vi "循环的使用.vi"() -> ()   [LabVIEW 2018]
panel:
  out "布尔":bool
  out "平均值":dbl
  # "创建一个VI，产生50个随机数，并采用循环结构求得这50个随机数的平均值，\n将平均值显示出来，再对平均值的范围进行判断，如果在0.6-0.9范围内，则\n点亮指示灯，否则知识点熄灭，并计算程序运行所消耗的时间。"
  # "20174080221\n王靖\n电子二班"
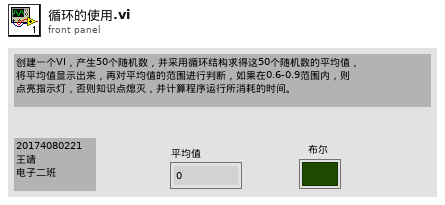
[diagram p1: front panel]
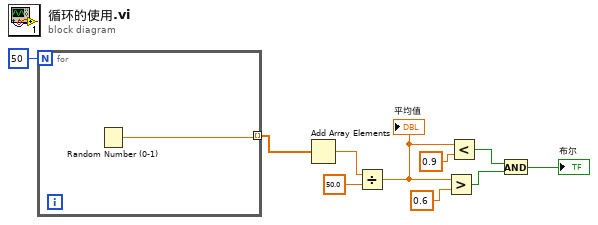
[diagram p0: block diagram]
diagram:
  n1 = for {
    N: 50 -> [_]
    tunnel: [w11] -> w9 mode=indexing
    n2 = Random Number (0-1) ("随机数(0-1)")() -> (number: 0 to 1=w11:dbl)
  }
  n3 = Add Array Elements(numeric array=w9) -> (sum=w8:dbl)
  n4 = Divide(x=w8, y=50.0) -> (x/y=w5:dbl)
  "平均值" <- w5
  n5 = Greater?(x=w5, y=0.6) -> (0:w3:bool)
  n6 = Less?(x=w5, y=0.9) -> (x < y?=w2:bool)
  n7 = And(x=w2, y=w3) -> (x .and. y?=→"布尔":bool)
